vi "))Channel.vi"(7 "This VI":refnum<vi>, 8 "Remove Queue":refnum<queue>, 9 "New Queue Depth":i32, 10 "channelOp":T3=enum."Close", 11 "channel in":T2) -> (1 "New Queue":refnum<queue>, 2 "Channel Data":T1, 3 "channel out":T2, 4 "Event Reg":refnum<event-registration>, 5 "This VI out":refnum<vi>)   [LabVIEW 2020, in "Flex.lvlib"]
uses:
  Flex.lvlib
  ChannelOp.ctl
  ))Channel.ctl
  Element.ctl
  Channel Data.ctl
  Element Info.ctl
  Event Data.ctl
  Queue Data.ctl
  Instantiate.vi
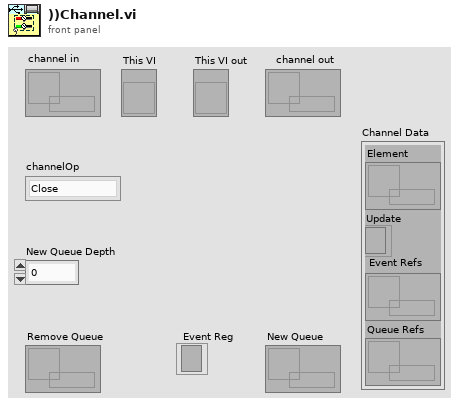
[diagram p1: front panel]
types:
  T1 = typedef "Flex.lvlib/Channel Data.ctl" = cluster{"Element":refnum<data-value>, "Update":refnum<k4>, "Event Refs":refnum<data-value>, "Queue Refs":refnum<data-value>}
  T2 = typedef "Flex.lvlib/))Channel.ctl" = refnum<queue>
  T3 = typedef "Flex.lvlib/ChannelOp.ctl" = enum16{"Get Refs", "Init", "Close", "Probe", "New Queue", "Remove Queue", "New Event"}
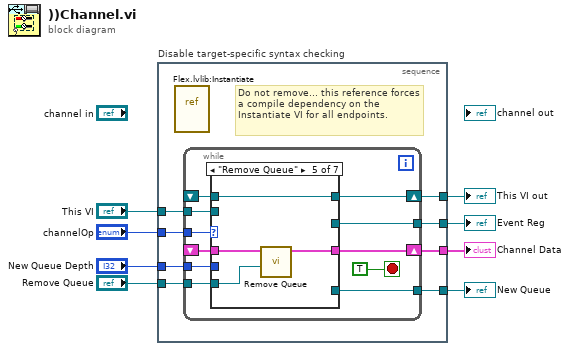
[diagram p0: block diagram]
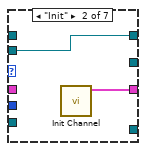
[diagram p3: hidden frame]
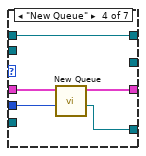
[diagram p5: hidden frame]
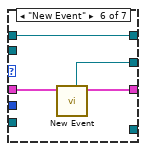
[diagram p6: hidden frame]
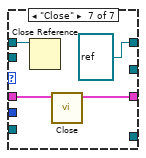
[diagram p7: hidden frame]
diagram:
  n1 = stacked-sequence "Disable target-specific syntax checking" {
    tunnel: "channelOp" -> [w16]
    tunnel: "This VI" -> [w15]
    tunnel: [w14] -> w6
    tunnel: "New Queue Depth" -> [w13]
    tunnel: [w12] -> w2
    tunnel: [w11] -> w4
    tunnel: "Remove Queue" -> [w10]
    tunnel: [w9] -> w3
    frame #0 {
      # "Do not remove... this reference forces a compile dependency on the Instantiate VI for all endpoints."
      n2 = vi-ref "Flex.lvlib:Instantiate.vi"() -> ()  [unwired: 1 out]
      n3 = while {
        tunnel: w16 -> [w25]
        shift-right: [w21] -> w11
        shift-left: _ -> [w27]
        shift-right: [w22] -> w14
        shift-left: _ -> [w23]
        tunnel: w15 -> [w24]
        tunnel: w13 -> [w20]
        tunnel: [w19] -> w12
        tunnel: w10 -> [w18]
        tunnel: [w17] -> w9
        stop <- TRUE stop-if-true
        n4 = case shown="\"Remove Queue\"" w25 {
          tunnel: [w28 w30 w32 w36 w40 w44 w47] -> w21
          tunnel: w27 -> [w28 _ w32 w37 w41 w45 w48]
          tunnel: w24 -> [_ w31 _ _ _ _ _]
          tunnel: [w29 w31 w33 w38 w42 w46 refnum<vi> refnum ("This VI")] -> w22
          tunnel: w23 -> [w29 _ w33 w38 w42 w46 w49]
          tunnel: w20 -> [_ _ _ w35 _ _ _]
          tunnel: [_ _ _ w34 _ _ _] -> w19
          tunnel: w18 -> [_ _ _ _ w39 _ _]
          tunnel: [_ _ _ _ _ w43 _] -> w17
          frame "Get Refs" {
          }
          frame "Init" {
            n5 = call "Init Channel.vi"() -> ("Channel Data"=w30:T1)  [unwired: 11 in]
          }
          frame "Probe" {
          }
          frame "New Queue" {
            n6 = call "New Queue.vi"("Depth"=w35, "Channel Data In"=w37) -> ("Queue"=w34:refnum<queue>, "Channel Data"=w36:T1)  [unwired: 8 in]
          }
          frame "Remove Queue" {
            n7 = call "Remove Queue.vi"("Queue"=w39, "Channel Data In"=w41) -> ("Channel Data"=w40:T1)  [unwired: 9 in]
          }
          frame "New Event" {
            n8 = call "New Event.vi"("Channel Data In"=w45) -> ("Channel Data"=w44:T1, "Event Reg"=w43:refnum<event-registration>)  [unwired: 9 in]
          }
          frame "Close" {
            n9 = Close Reference(reference=w49) -> ()  [unwired: 1 in, 1 out]
            n10 = call "Close.vi"("Channel Data In"=w48) -> ("Channel Data"=w47:T1)  [unwired: 10 in]
          }
        }
      }
    }
  }
  "This VI out" <- w6
  "Channel Data" <- w4
  "Event Reg" <- w3
  "New Queue" <- w2
